vi "FVIR_LDO_Inficon.vi"(8 "error in":errorcluster, 10 "Remote IP Address":string="192.168.1.32", 11 "Message Queues":T1) -> (0 "error out":errorcluster)   [LabVIEW 2020]
uses:
  Message Queue/All Message Queues.ctl
  Message Queue/Message Cluster.ctl
  Drivers/Inficon Transmitter/Type Definitions/Inficon Data.ctl
  Message Queue/Enqueue Message (Single).vi
  <vilib>/NI/Modbus Library/API/Wrapper/Create TCP Master.vi
  <vilib>/NI/Modbus Library/API/Master/Modbus Master.lvclass
  Message Queue/Message Queue.lvlib
  <vilib>/NI/Modbus Library/API/Wrapper/API Main.lvlib
panel:
  # "NG Inficon: 192.168.1.32\nLP Inficon: 192.168.1.33"
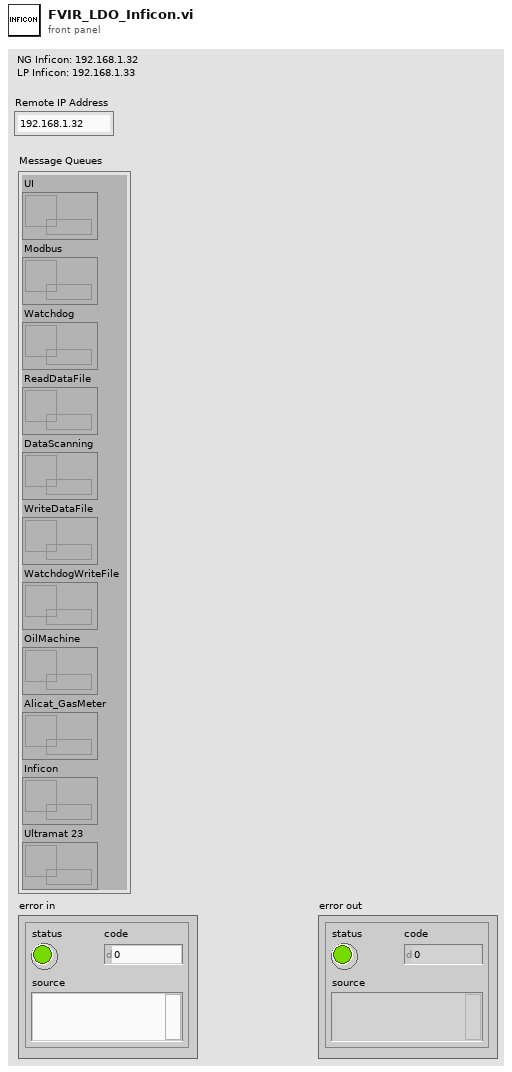
[diagram p1: front panel]
types:
  T1 = typedef "Message Queue.lvlib/All Message Queues.ctl" = cluster{"UI":refnum<queue>, "Modbus":refnum<queue>, "Watchdog":refnum<queue>, "ReadDataFile":refnum<queue>, "DataScanning":refnum<queue>, "WriteDataFile":refnum<queue>, "WatchdogWriteFile":refnum<queue>, "OilMachine":refnum<queue>, "Alicat_GasMeter":refnum<queue>, "Inficon":refnum<queue>, "Ultramat 23":refnum<queue>}
  T2 = typedef "Inficon Data.ctl" = cluster{"Gross Heating Value, Vol (Real, Dry)":dbl, "Nitrogen Component Normalized Mole % (Dry)":dbl, "Methane Component Normalized Mole % (Dry)":dbl, "Carbon Dioxide Component Normalized Mole % (Dry)":dbl, "Ethane Component Normalized Mole % (Dry)":dbl, "Propane Component Normalized Mole % (Dry)":dbl, "i-Pentane Component Normalized Mole % (Dry)":dbl, "i-Butane Component Normalized Mole % (Dry)":dbl, "n-Butane Component Normalized Mole % (Dry)":dbl, "n-Pentane Component Normalized Mole % (Dry)":dbl, "Hexane Component Normalized Mole % (Dry)":dbl, "Heptane Component Normalized Mole % (Dry)":dbl, "Gross Wobbe Index, Real(Dry)":dbl, "Relative Density, Real(Dry)":dbl, "Propylene Component Normalized Mole % (Dry)":dbl, "C4 Olefins Component Normalized Mole % (Dry)":dbl, "Water Component Normalized Mole % (Dry)":dbl}
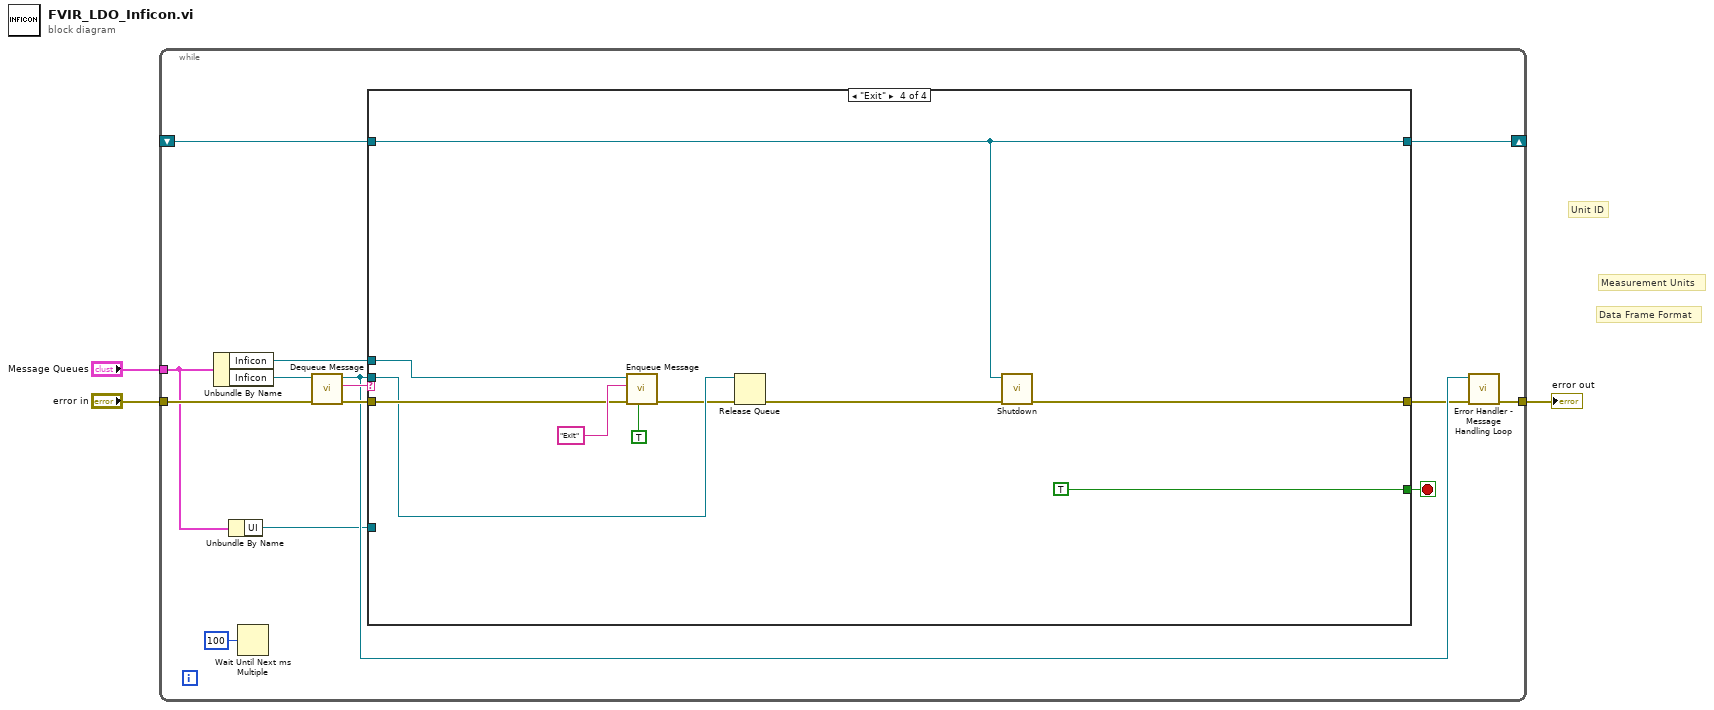
[diagram p0: block diagram]
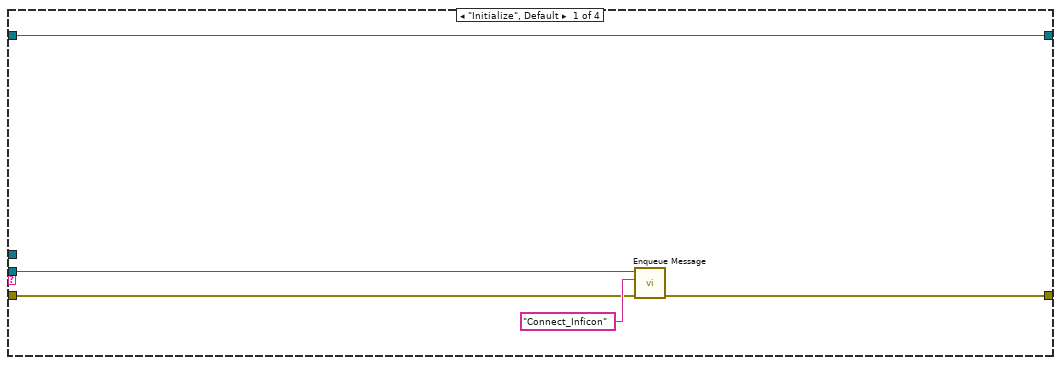
[diagram p2: hidden frame]
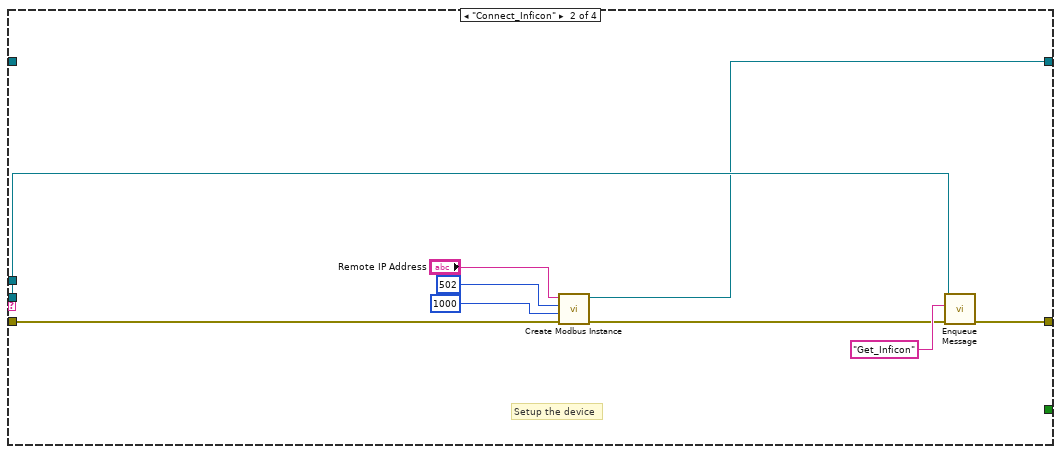
[diagram p3: hidden frame]
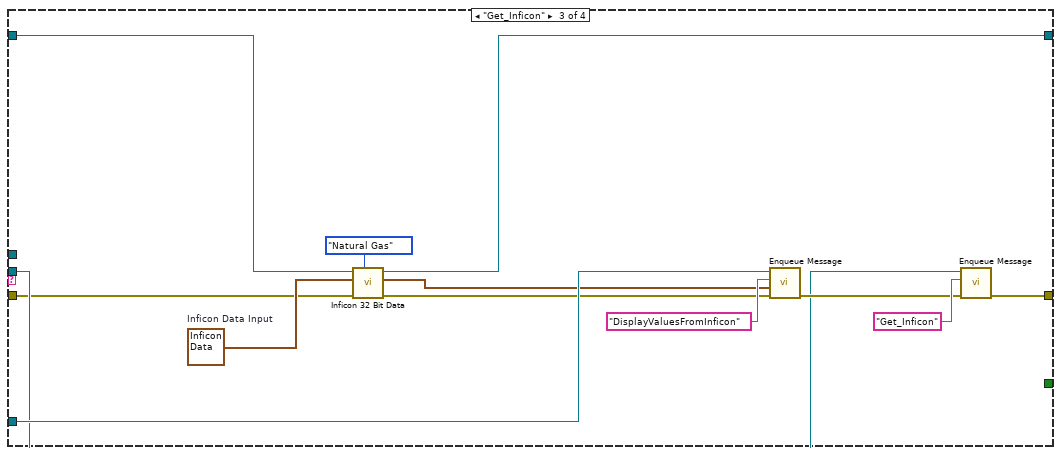
[diagram p4: hidden frame]
diagram:
  # "Unit ID"
  # "Data Frame Format"
  # "Measurement Units"
  n1 = while {
    tunnel: "Message Queues" -> [w7]
    tunnel: "error in" -> [w16]
    tunnel: [w10] -> w1
    shift-right: [w5] -> _
    shift-left: _ -> [w4]
    stop <- w13 stop-if-true
    n2 = Unbundle By Name(w7) -> ("Inficon"=w12:refnum<queue>, "Inficon"=w17:refnum<queue>)
    n3 = Unbundle By Name(w7) -> ("UI"=w6:refnum<queue>)
    n4 = Wait Until Next ms Multiple(millisecond multiple=u32 100) -> ()  [unwired: 1 out]
    n5 = call "Dequeue Message.vi"("error in (no error)"=w16, "Message Queue"=w17) -> ("error out"=w14:errorcluster, "Message"=w15:string, "dup Message Queue"=w11:refnum<queue>)  [unwired: 6 in, 1 out]
    n6 = case shown="\"Exit\"" w15 {
      tunnel: w14 -> [w21 w24 w36 w50]
      tunnel: [w20 w30 w40 w46] -> w9
      tunnel: [_ _ _ TRUE] -> w13
      tunnel: w12 -> [_ _ _ w51]
      tunnel: w11 -> [w19 w29 w39 w49]
      tunnel: w6 -> [_ _ w43 _]
      tunnel: [w18 w23 w37 w45] -> w5
      tunnel: w4 -> [w18 _ w32 w45]
      frame "Initialize", Default {
        n7 = call-poly "Enqueue Message.vi"("error in (no error)"=w21, "Message"="Connect_Inficon", "Message Queue"=w19) -> ("error out"=w20:errorcluster)  [unwired: 7 in, 1 out]
      }
      frame "Connect_Inficon" {
        # "Setup the device"
        n8 = call-poly <vilib>:"Create Modbus Instance.vi"("error in"=w24, "connect timeout ms"=1000, "port (502)"=u16 502, "address"="Remote IP Address") -> ("error out"=w25:errorcluster, "TCP master instance"=w23:refnum<class "Modbus Master.lvclass">)  [unwired: 6 in]
        n9 = call-poly "Enqueue Message.vi"("error in (no error)"=w25, "Message"="Get_Inficon", "Message Queue"=w29) -> ("error out"=w30:errorcluster)  [unwired: 7 in, 1 out]
      }
      frame "Get_Inficon" {
        w38 = T2 {"Gross Heating Value, Vol (Real, Dry)"=0.0, "Nitrogen Component Normalized Mole % (Dry)"=0.0, "Methane Component Normalized Mole % (Dry)"=0.0, "Carbon Dioxide Component Normalized Mole % (Dry)"=0.0, "Ethane Component Normalized Mole % (Dry)"=0.0, "Propane Component Normalized Mole % (Dry)"=0.0, "i-Pentane Component Normalized Mole % (Dry)"=0.0, "i-Butane Component Normalized Mole % (Dry)"=0.0, "n-Butane Component Normalized Mole % (Dry)"=0.0, "n-Pentane Component Normalized Mole % (Dry)"=0.0, "Hexane Component Normalized Mole % (Dry)"=0.0, "Heptane Component Normalized Mole % (Dry)"=0.0, "Gross Wobbe Index, Real(Dry)"=0.0, "Relative Density, Real(Dry)"=0.0, "Propylene Component Normalized Mole % (Dry)"=0.0, "C4 Olefins Component Normalized Mole % (Dry)"=0.0, "Water Component Normalized Mole % (Dry)"=0.0}  # Inficon Data Input
        n10 = call "Inficon 32 Bit Data.vi"("Gas Type"=enum16{"Natural Gas", "Propane Gas"}."Natural Gas", "Error In"=w36, "Inficon Data Input"=w38, "Modbus master in"=w32) -> ("Error Out"=w35:errorcluster, "Inficon Data Output"=w34:T2, "Modbus master out"=w37:refnum<class "Modbus Master.lvclass">)  [unwired: 4 in, 1 out]
        n11 = call-poly "Enqueue Message.vi"("error in (no error)"=w35, "Message Data"=w34, "Message"="DisplayValuesFromInficon", "Message Queue"=w43) -> ("error out"=w41:errorcluster)  [unwired: 6 in, 1 out]
        n12 = call-poly "Enqueue Message.vi"("error in (no error)"=w41, "Message"="Get_Inficon", "Message Queue"=w39) -> ("error out"=w40:errorcluster)  [unwired: 7 in, 1 out]
      }
      frame "Exit" {
        n13 = call-poly "Enqueue Message.vi"("Priority Message? (F)"=TRUE, "error in (no error)"=w50, "Message"="Exit", "Message Queue"=w51) -> ("error out"=w48:errorcluster)  [unwired: 6 in, 1 out]
        n14 = Release Queue(queue=w49, error in (no error)=w48) -> (error out=w47:errorcluster)  [unwired: 1 in, 2 out]
        n15 = call-dynamic "Shutdown.vi"("error in"=w47, "Modbus master in"=w45) -> ("error out"=w46:errorcluster)  [unwired: 9 in]
      }
    }
    n16 = call "Error Handler - Message Handling Loop.vi"("error in (no error)"=w9, "Message Queue"=w11) -> ("dup error in"=w10:errorcluster)  [unwired: 8 in, 1 out]
  }
  "error out" <- w1
